vi "TL Motor MoveRelative.vi"() -> ()   [LabVIEW 2021]
doc: "Shows how to perform a relative motor move."
panel:
  in  "MG17Motor":refnum<k7>(container)
  in  "Stop":bool
  in  "Set Rel Move Size":bool
  in  "Rel Move Size":dbl=1.0 min=-10.0 max=10.0 format="%.2f"
  in  "Move Relative":bool
  in  "Home":bool
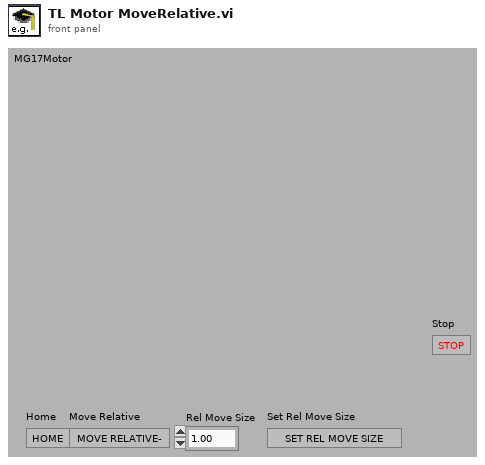
[diagram p1: front panel]
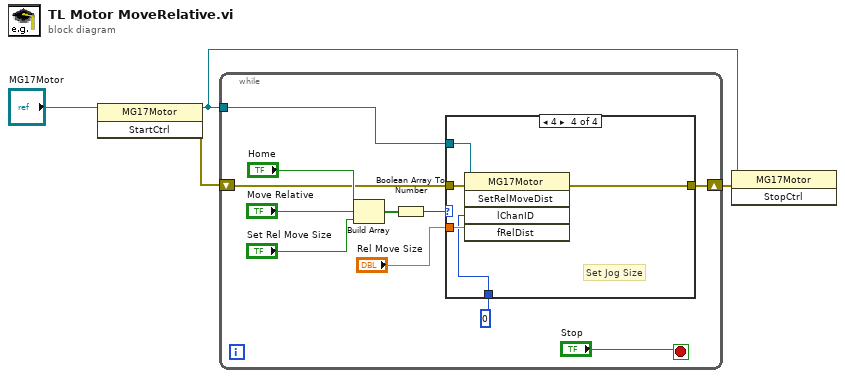
[diagram p0: block diagram]
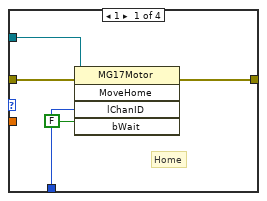
[diagram p2: hidden frame]
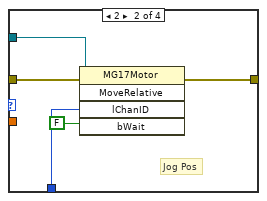
[diagram p3: hidden frame]
diagram:
  n1 = invoke class="MG17Motor" method="StartCtrl"(reference="MG17Motor") -> (reference out=w4:refnum<k7>, error out=w3:errorcluster)  [unwired: 2 in, 1 out]
  n2 = while {
    shift-left: w3 -> [w8]
    shift-right: [w9] -> w2
    tunnel: w4 -> [w13]
    stop <- "Stop" stop-if-true
    n3 = Build Array("Home", "Move Relative", "Set Rel Move Size") -> (w5:bool[])
    n4 = Boolean Array To Number(Boolean array=w5) -> (number=w6:u32)
    n5 = case shown="4" w6 {
      tunnel: w13 -> [w20 w25 _ w31]
      tunnel: 0 ("lChanID") -> [w19 w24 _ w27]
      tunnel: "Rel Move Size" -> [_ _ _ w30]
      tunnel: [w18 w23 w26 w28] -> w9
      tunnel: w8 -> [w17 w21 w26 w29]
      frame 1 {
        # "Home"
        n6 = invoke class="MG17Motor" method="MoveHome"(reference=w20, error in=w17, "lChanID"=w19, "bWait"=FALSE) -> (error out=w18:errorcluster)  [unwired: 1 in, 4 out]
      }
      frame 2 {
        # "Jog Pos"
        n7 = invoke class="MG17Motor" method="MoveRelative"(reference=w25, error in=w21, "lChanID"=w24, "bWait"=FALSE) -> (error out=w23:errorcluster)  [unwired: 1 in, 4 out]
      }
      frame Default {
      }
      frame 4 {
        # "Set Jog Size"
        n8 = invoke class="MG17Motor" method="SetRelMoveDist"(reference=w31, error in=w29, "lChanID"=w27, "fRelDist"=w30) -> (error out=w28:errorcluster)  [unwired: 1 in, 4 out]
      }
    }
  }
  n9 = invoke class="MG17Motor" method="StopCtrl"(reference=w4, error in=w2) -> ()  [unwired: 1 in, 3 out]
